vi "test-file_transfer_engine.vi"() -> ()   [LabVIEW 2017, in "labview-standard-library.lvlib"]
uses:
  labview-standard-library.lvlib
panel:
  in  "Array":path[](array[path])
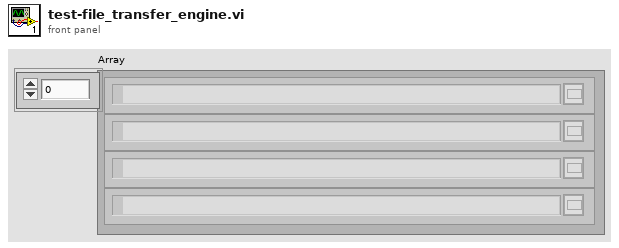
[diagram p1: front panel]
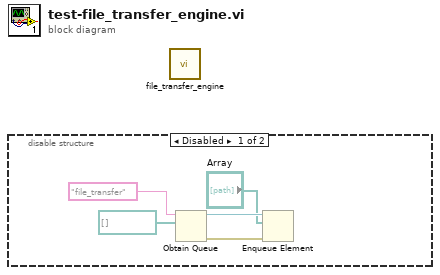
[diagram p0: block diagram]
diagram:
  n1 = disable-structure shown="Disabled" {
    frame Disabled {
      n2 = Obtain Queue(name (unnamed)="file_transfer", element data type=path[] []) -> (queue out=w3:refnum<queue>, error out=w2:errorcluster)  [unwired: 3 in, 1 out]
      n3 = Enqueue Element(queue=w3, element="Array", error in (no error)=w2) -> ()  [unwired: 1 in, 3 out]
    }
    frame Enabled {
    }
  }
  n4 = call "file_transfer_engine.vi"() -> ()  [unwired: 12 in]
